vi "IMU_Single_Write_Data.vi"(7 "Command Selection":u16(ring) items=["MSP_IDENT", "MSP_STATUS", "MSP_RAW_IMU", "MSP_RAW_GPS", "MSP_ATTITUDE", "MSP_ALTITUDE", "MSP_ACC_CALIBRATION", "MSP_MAG_CALIBRATION"], 8 "error in (no error)":errorcluster caption="Fehler (Eingang, kein Fehler)", 11 "VISA resource name IN":refnum<visa-resource-name>) -> (0 "error out":errorcluster caption="Fehler (Ausgang)", 3 "VISA resource name OUT":refnum<visa-resource-name>)   [LabVIEW 2017]
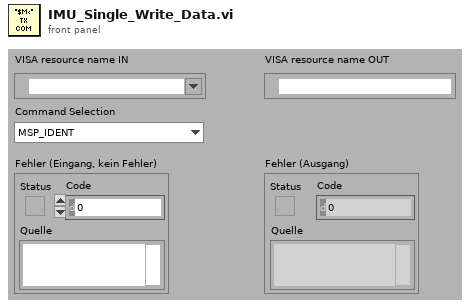
[diagram p1: front panel]
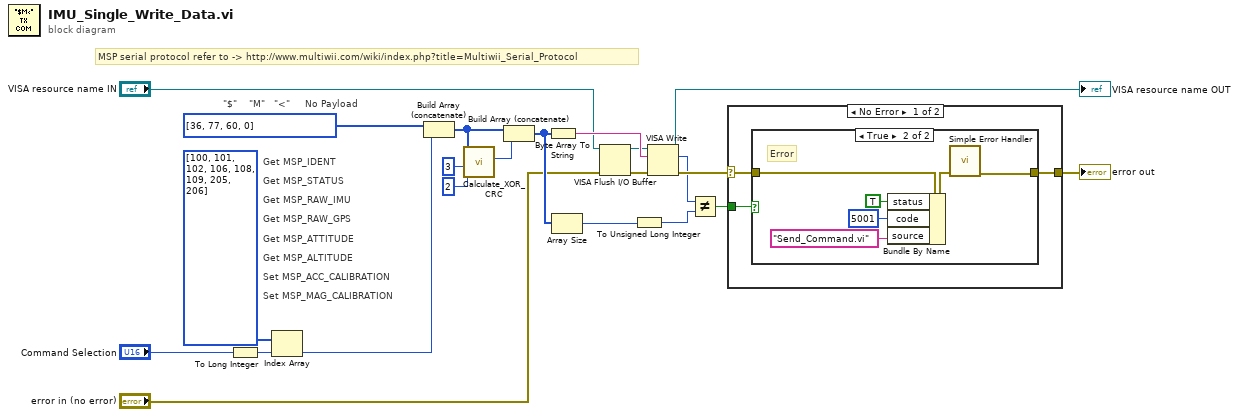
[diagram p0: block diagram]
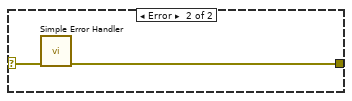
[diagram p3: hidden frame]
diagram:
  # "MSP serial protocol refer to -> http://www.multiwii.com/wiki/index.php?title=Multiwii_Serial_Protocol"
  # "\"$\"    \"M\"   \"<\"     No Payload"
  # "Set MSP_MAG_CALIBRATION"
  # "Set MSP_ACC_CALIBRATION"
  # "Get MSP_ALTITUDE"
  # "Get MSP_ATTITUDE"
  # "Get MSP_RAW_GPS"
  # "Get MSP_RAW_IMU"
  # "Get MSP_STATUS"
  # "Get MSP_IDENT"
  n1 = To Long Integer(number="Command Selection") -> (32bit integer=w1:i32)
  n2 = Index Array(array=u8[] [100, 101, 102, 106, 108, 109, 205, 206], index=w1) -> (element=w18:u8)
  n3 = Build Array (concatenate)(u8[] [36, 77, 60, 0], w18) -> (w17:u8[])
  n4 = call "Calculate_XOR_CRC.vi"("No. of Bytes for Calculation"=2, "Start Position (Byte)"=3, "U8 Byte Array"=w17) -> ("CRC"=w16:u8)  [unwired: 8 in]
  n5 = Build Array (concatenate)(w17, w16) -> (w12:u8[])
  n6 = Byte Array To String(unsigned byte array=w12) -> (string=w13:string)
  n7 = Array Size(array=w12) -> (size(s)=w14:i32)
  n8 = VISA Flush I/O Buffer(VISA resource name="VISA resource name IN", error in (no error)="error in (no error)") -> (VISA resource name out=w2:refnum<visa-resource-name>, error out=w5:errorcluster)  [unwired: 1 in]
  n9 = To Unsigned Long Integer(number=w14) -> (unsigned 32bit integer=w11:u32)
  n10 = VISA Write(VISA resource name=w2, write buffer=w13, error in (no error)=w5) -> (VISA resource name out=→"VISA resource name OUT":refnum<visa-resource-name>, return count=w7:u32, error out=w9:errorcluster)
  n11 = Not Equal?(x=w7, y=w11) -> (x != y?=w8:bool)
  n12 = case shown="No Error" w9 {
    selector: w9 -> [w24 w34]
    tunnel: w8 -> [w25 _]
    tunnel: [w23 w33] -> w6
    frame No Error {
      n13 = case shown="True" w25 {
        tunnel: w24 -> [w26 w32]
        tunnel: [w26 w27] -> w23
        frame False {
          # "no Error"
        }
        frame True {
          # "Error"
          n14 = Bundle By Name(cluster=w32, "status"=TRUE, "code"=5001, "source"="Send_Command.vi") -> (w29:errorcluster)
          n15 = call <vilib>:"Simple Error Handler.vi"("error in (no error)"=w29) -> ("error out"=w27:errorcluster)  [unwired: 4 in, 4 out]
        }
      }
    }
    frame Error {
      n16 = call <vilib>:"Simple Error Handler.vi"("error in (no error)"=w34) -> ("error out"=w33:errorcluster)  [unwired: 4 in, 4 out]
    }
  }
  "error out" <- w6
